vi "PID Aim.vi"   [LabVIEW 2015]
uses:
  Vision/Vision Global.vi
  <vilib>/addons/control/pid/pid.llb/PID (DBL).vi
  <vilib>/addons/control/pid/NI_PID_pid.lvlib
types:
  T1 = cluster{"proportional gain (Kc)":dbl, "integral time (Ti, min)":dbl, "derivative time (Td, min)":dbl}
  T2 = cluster{"Distance (ft)":dbl, "Center":cluster{dbl, dbl}, "Normalized Rect":cluster{"Numeric":dbl, "Numeric 2":dbl, "Numeric 3":dbl, "Numeric 5":dbl}}[]
  T3 = cluster{"Distance (ft)":dbl, "Center":cluster{dbl, dbl}, "Normalized Rect":cluster{"Numeric":dbl, "Numeric 2":dbl, "Numeric 3":dbl, "Numeric 5":dbl}}
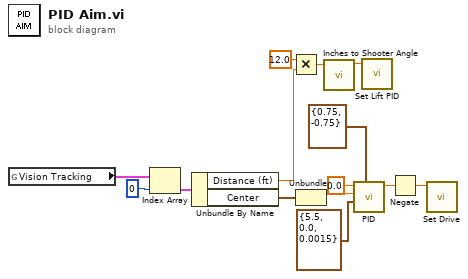
[diagram p0: block diagram]
diagram:
  n1 = global read "Vision Global.vi" "Vision Tracking"() -> (w12:T2)
  n2 = Index Array(array=w12, index=0) -> (element=w13:T3)
  n3 = Unbundle By Name(w13) -> ("Distance (ft)"=w4:dbl, "Center"=w11:cluster{dbl, dbl})
  n4 = Multiply(x=12.0, y=w4) -> (x*y=w2:dbl)
  n5 = Unbundle(w11) -> (w9:dbl)  [unwired: 1 out]
  n6 = call "Inches to Shooter Angle.vi"("distance (in)"=w2) -> ("arm angle"=w1:dbl)  [unwired: 10 in]
  n7 = call-poly <vilib>:"PID.vi"("output range"=cluster{"output high":dbl, "output low":dbl} {"output high"=0.75, "output low"=-0.75}, "PID gains"=T1 {"proportional gain (Kc)"=5.5, "integral time (Ti, min)"=0.0, "derivative time (Td, min)"=0.0015}, "process variable"=w9, "setpoint"=0.0) -> ("output"=w10:dbl)  [unwired: 6 in, 1 out]
  n8 = call "Set Lift PID.vi"("setpoint"=w1) -> ()  [unwired: 11 in]
  n9 = Negate(x=w10) -> (-x=w7:dbl)
  n10 = call "Set Drive.vi"("X axis value"=w7) -> ()  [unwired: 11 in]
